vi "Remove Duplicates from 1D Array.vi"(0 "Input Array":string[](array[string])) -> (1 "Output Array":string[](array[string]), 2 "indices of removed elements":i32[](array[numeric]))   [LabVIEW 2018, in "Numeric Data Type.lvclass"]
doc: "<b> </b> <b> </b>\n©2013, Q Software Innovations, LLC.\n\nWritten in National Instruments LabVIEW™ 2013.\n\nAuthored by Quentin Alldredge\nQ@qsoftwareinnovations.com\nwww.qsoftwareinnovations.com\n\nAll rights reserved."
uses:
  Numeric Data Type.lvclass
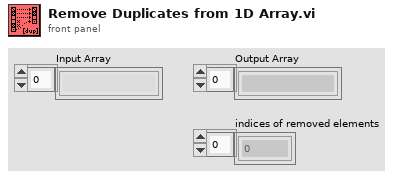
[diagram p1: front panel]
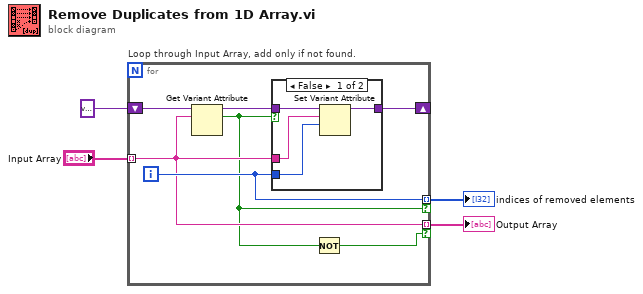
[diagram p0: block diagram]
diagram:
  n1 = for "Loop through Input Array, add only if not found." {
    shift-right: [w11] -> _
    shift-left: variant -> [w10]
    tunnel: "Input Array" -> [w7] mode=indexing
    tunnel: [w8] -> w4 mode=indexing if=w6
    tunnel: [w7] -> w1 mode=indexing if=w5
    i -> [w8]
    n2 = Get Variant Attribute(Variant=w10, name=w7) -> (duplicate Variant=w9:variant, found=w6:bool)  [unwired: 2 in, 2 out]
    n3 = case shown="False" w6 {
      tunnel: [w15 w16] -> w11
      tunnel: w7 -> [w14 _]
      tunnel: w9 -> [w13 w16]
      tunnel: w8 -> [w12 _]
      frame False {
        n4 = Set Variant Attribute(Variant=w13, name=w14, value=w12) -> (Variant out=w15:variant)  [unwired: 1 in, 2 out]
      }
      frame True {
      }
    }
    n5 = Not(x=w6) -> (.not. x?=w5:bool)
  }
  "indices of removed elements" <- w4
  "Output Array" <- w1
